vi "Search Or Add Frame.vi"(10 "Detection Frame In 3":T1 {"robots_blue"."height" format="%+4.3f"; "robots_blue"."pixel_y" format="%+4.3f"; "robots_blue"."pixel_x" format="%+4.3f"; "robots_blue"."orientation" format="%+4.3f"; "robots_blue"."y" format="%+4.3f"; "robots_blue"."confidence" format="%4.3f"; "robots_blue"."x" format="%+4.3f"; "robots_yellow"."height" format="%+4.3f"; "robots_yellow"."pixel_y" format="%+4.3f"; "robots_yellow"."pixel_x" format="%+4.3f"; "robots_yellow"."orientation" format="%+4.3f"; "robots_yellow"."y" format="%+4.3f"; "robots_yellow"."confidence" format="%4.3f"; "robots_yellow"."x" format="%+4.3f"}, 11 "Detection Frame In 4":T1[](array[typedef]) {"robots_blue"."height" format="%+4.3f"; "robots_blue"."pixel_y" format="%+4.3f"; "robots_blue"."pixel_x" format="%+4.3f"; "robots_blue"."orientation" format="%+4.3f"; "robots_blue"."y" format="%+4.3f"; "robots_blue"."confidence" format="%4.3f"; "robots_blue"."x" format="%+4.3f"; "robots_yellow"."height" format="%+4.3f"; "robots_yellow"."pixel_y" format="%+4.3f"; "robots_yellow"."pixel_x" format="%+4.3f"; "robots_yellow"."orientation" format="%+4.3f"; "robots_yellow"."y" format="%+4.3f"; "robots_yellow"."confidence" format="%4.3f"; "robots_yellow"."x" format="%+4.3f"}) -> (3 "Detection Frame In 2":T1[](array[typedef]) {"robots_blue"."height" format="%+4.3f"; "robots_blue"."pixel_y" format="%+4.3f"; "robots_blue"."pixel_x" format="%+4.3f"; "robots_blue"."orientation" format="%+4.3f"; "robots_blue"."y" format="%+4.3f"; "robots_blue"."confidence" format="%4.3f"; "robots_blue"."x" format="%+4.3f"; "robots_yellow"."height" format="%+4.3f"; "robots_yellow"."pixel_y" format="%+4.3f"; "robots_yellow"."pixel_x" format="%+4.3f"; "robots_yellow"."orientation" format="%+4.3f"; "robots_yellow"."y" format="%+4.3f"; "robots_yellow"."confidence" format="%4.3f"; "robots_yellow"."x" format="%+4.3f"})   [LabVIEW 2017]
uses:
  SSL Detection Frame.ctl
  SSL Detection Robot.ctl
  <vilib>/Analysis/Matrix/Datatypes/RealMatrix.ctl
  SSL Detection Ball.ctl
  <vilib>/Analysis/Matrix/NI_Matrix.lvlib
panel:
  in  "CamerasToIgnore":dbl[](array[numeric])=[-1.0]
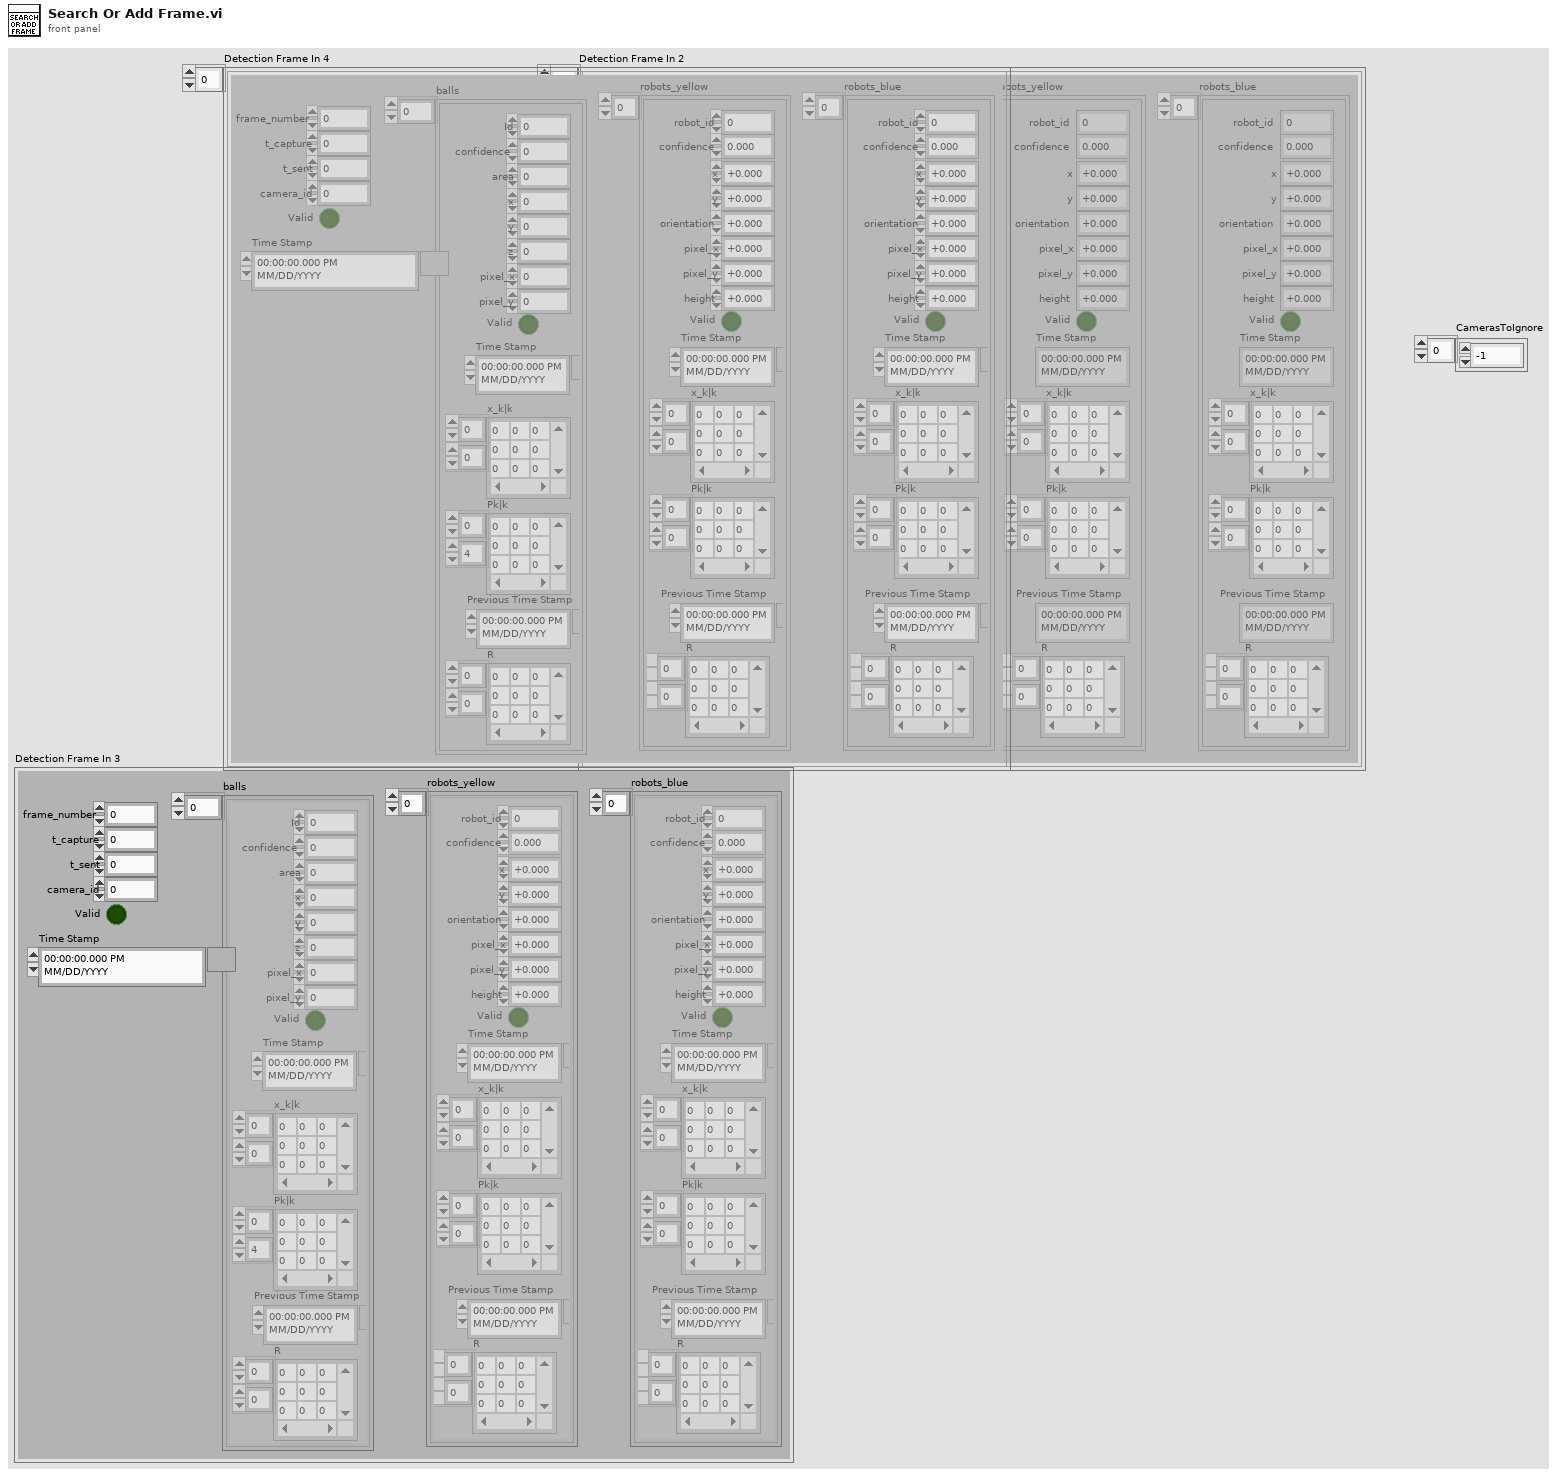
[diagram p1: front panel]
types:
  T1 = typedef "SSL Detection Frame.ctl" = cluster{"frame_number":u32, "t_capture":dbl, "t_sent":dbl, "camera_id":u32, "robots_yellow":T2[], "robots_blue":T2[], "balls":T4[], "Valid":bool, "Time Stamp":timestamp}
  T2 = typedef "SSL Detection Robot.ctl" = cluster{"x":sgl, "robot_id":u32, "confidence":sgl, "y":sgl, "orientation":sgl, "pixel_x":sgl, "pixel_y":sgl, "height":sgl, "Valid":bool, "Time Stamp":timestamp, "x_k|k":T3, "Pk|k":T3, "Previous Time Stamp":timestamp, "R":T3}
  T3 = typedef "NI_Matrix.lvlib/RealMatrix.ctl" = dbl[][]
  T4 = typedef "SSL Detection Ball.ctl" = cluster{"x":sgl, "area":u32, "confidence":sgl, "y":sgl, "z":sgl, "pixel_x":sgl, "pixel_y":sgl, "Valid":bool, "Time Stamp":timestamp, "x_k|k":T3, "Pk|k":T3, "Id":u32, "Previous Time Stamp":timestamp, "R":T3}
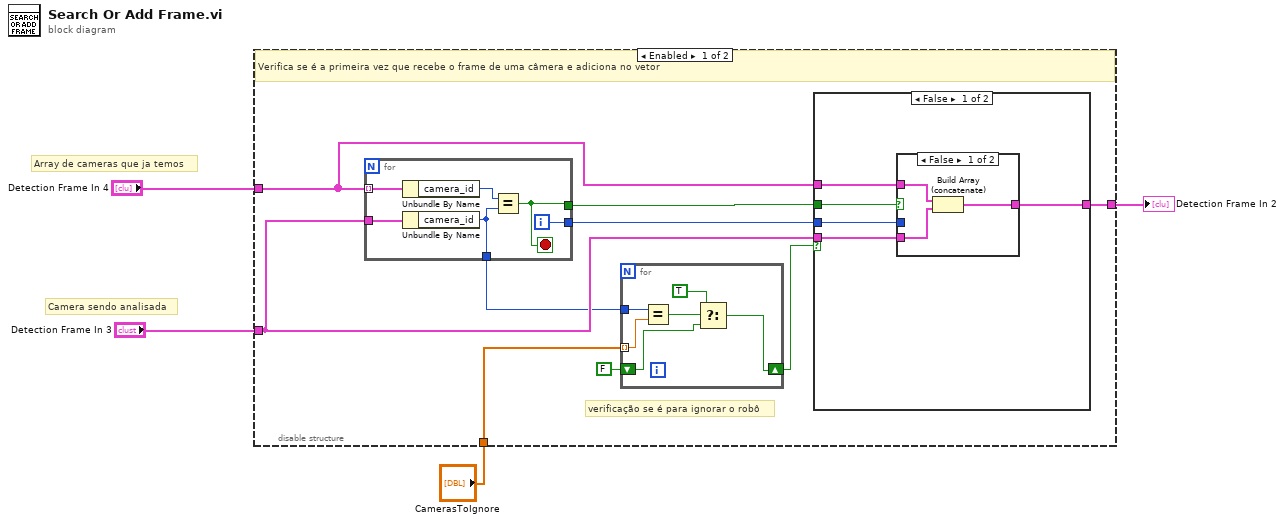
[diagram p0: block diagram]
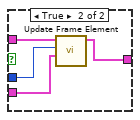
[diagram p2: hidden frame]
diagram:
  # "Camera sendo analisada"
  # "Array de cameras que ja temos"
  n1 = disable-structure "Diagram Disable Structure" shown="Enabled" {
    disable-tunnel: "Detection Frame In 4" -> [w12 _]
    disable-tunnel: "Detection Frame In 3" -> [w10 _]
    disable-tunnel: [w9 _] -> w4
    disable-tunnel: "CamerasToIgnore" -> [w7 _]
    frame Enabled {
      # "verificação se é para ignorar o robô"
      # "Verifica se é a primeira vez que recebe o frame de uma câmera e adiciona no vetor"
      n2 = for {
        tunnel: w12 -> [w38] mode=indexing
        tunnel: w10 -> [w37]
        tunnel: [w35] -> w13
        tunnel: [w34] -> w11
        tunnel: [w33] -> w8
        i -> [w34]
        stop <- w35 stop-if-true
        n3 = Unbundle By Name(w38) -> ("camera_id"=w36:u32)
        n4 = Unbundle By Name(w37) -> ("camera_id"=w33:u32)
        n5 = Equal?(x=w36, y=w33) -> (x = y?=w35:bool)
      }
      n6 = for {
        tunnel: w8 -> [w32]
        tunnel: w7 -> [w31] mode=indexing
        shift-right: [w28] -> w5
        shift-left: FALSE -> [w27]
        n7 = Equal?(x=w32, y=w31) -> (x = y?=w30:bool)
        n8 = Select(t=TRUE, s=w30, f=w27) -> (s? t:f=w28:bool)
      }
      n9 = case shown="False" w5 {
        tunnel: w13 -> [w18 _]
        tunnel: w12 -> [w17 w26]
        tunnel: w11 -> [w16 _]
        tunnel: w10 -> [w15 _]
        tunnel: [w14 w26] -> w9
        frame False {
          n10 = case shown="False" w18 {
            tunnel: w17 -> [w21 w25]
            tunnel: w15 -> [w19 w23]
            tunnel: [w20 w22] -> w14
            tunnel: w16 -> [_ w24]
            frame False {
              n11 = Build Array (concatenate)(w21, w19) -> (w20:T1[])
            }
            frame True {
              n12 = call "Update Frame Element.vi"("Detection Frame In in"=w23, "Numeric"=w24, "Detection Frame In 3"=w25) -> ("Detection Frame In out"=w22:T1[])  [unwired: 8 in]
            }
          }
        }
        frame True {
        }
      }
    }
    frame Disabled {
    }
  }
  "Detection Frame In 2" <- w4
